vi "单道符合.vi"() -> ()   [LabVIEW 2014]
panel:
  in  "清零":bool
  in  "开始":bool
  out "状态":enum16{"初始化", "空闲", "配置", "读取", "退出"}(ring)
  out "coincnt":i32
  out "Bcnt":i32
  out "Acnt":i32
  in  "单道2道宽":u16=3000
  in  "单道2阈值电压":u16=100
  in  "单道1道宽":u16=3000
  in  "单道1阈值电压":u16=100
  in  "runtime(秒)":u16=10
  in  "cointime3":u16
  in  "cointime2":u16
  in  "cointime1":u16
  in  "退出":bool
  in  "读取":bool
  in  "配置":bool
  in  "初始状态":enum16{"初始化", "空闲", "配置", "读取", "退出"}(ring)
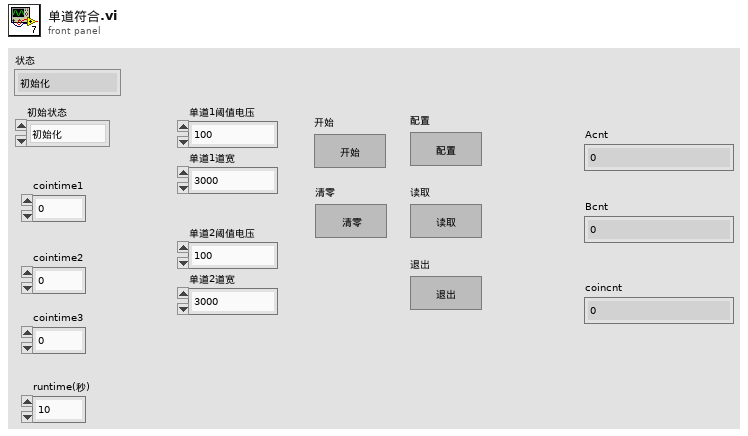
[diagram p1: front panel]
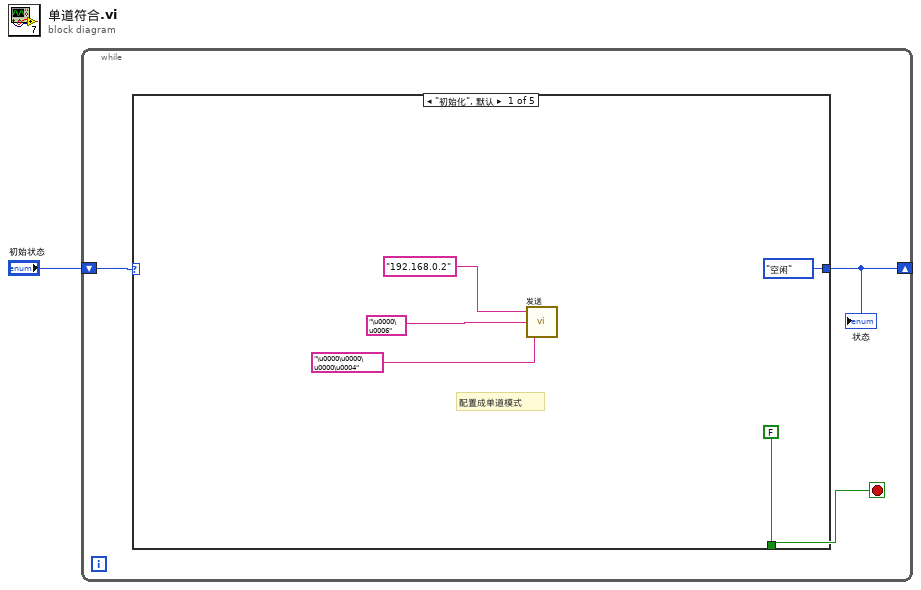
[diagram p0: block diagram]
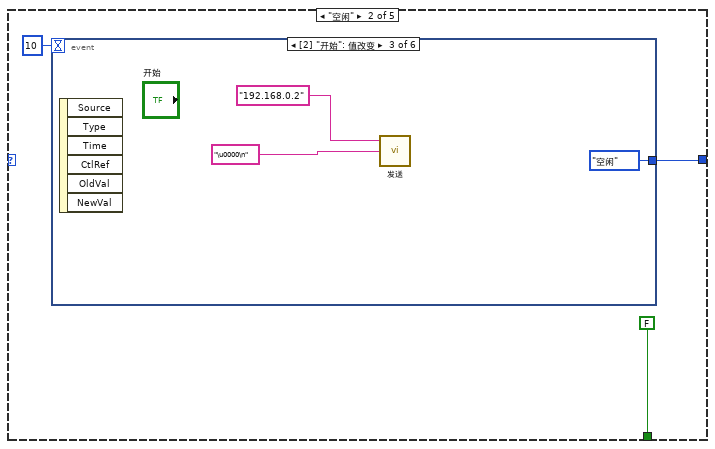
[diagram p2: hidden frame]
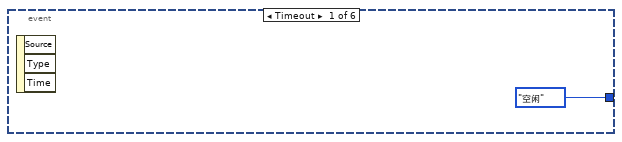
[diagram p3: hidden frame]
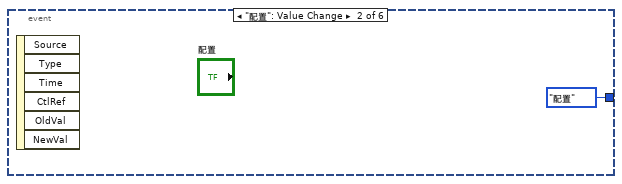
[diagram p4: hidden frame]
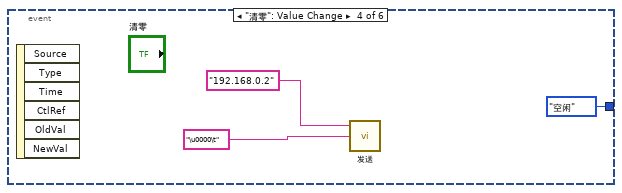
[diagram p5: hidden frame]
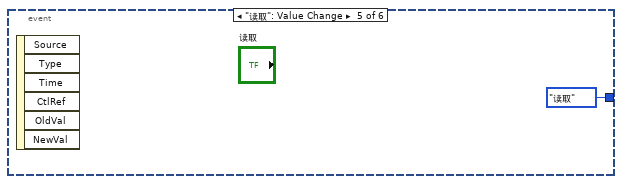
[diagram p6: hidden frame]
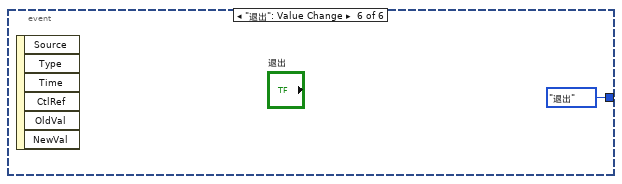
[diagram p7: hidden frame]
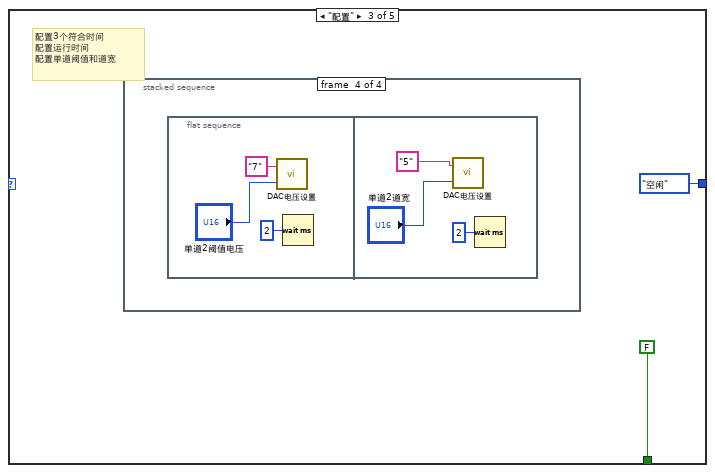
[diagram p8: hidden frame]
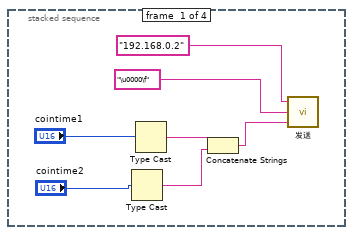
[diagram p9: hidden frame]
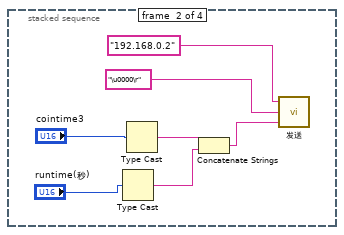
[diagram p10: hidden frame]
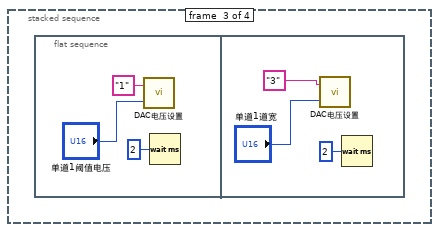
[diagram p11: hidden frame]
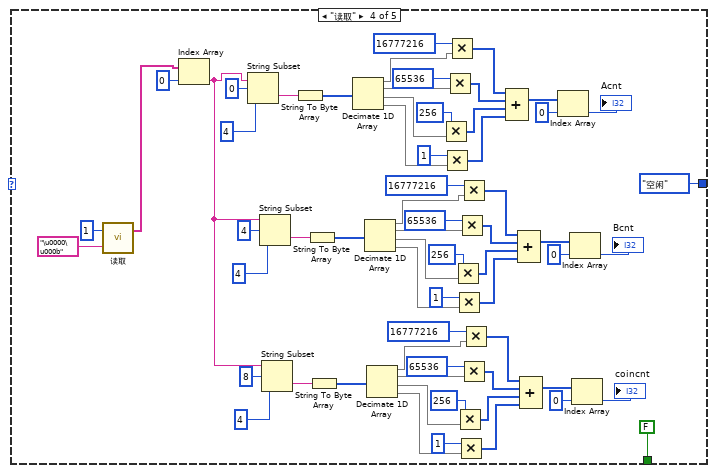
[diagram p12: hidden frame]
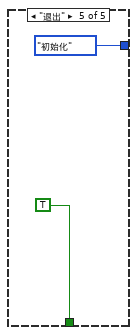
[diagram p13: hidden frame]
diagram:
  n1 = while {
    shift-right: [w3] -> _
    shift-left: "初始状态" -> [w4]
    stop <- w2 stop-if-true
    n2 = case shown="\"初始化\", 默认" w4 {
      tunnel: [enum16{"初始化", "空闲", "配置", "读取", "退出"}."空闲" ("初始状态") w11 enum16{"初始化", "空闲", "配置", "读取", "退出"}."空闲" ("初始状态") enum16{"初始化", "空闲", "配置", "读取", "退出"}."空闲" ("初始状态") enum16{"初始化", "空闲", "配置", "读取", "退出"}."初始化" ("初始状态")] -> w3
      tunnel: [FALSE FALSE FALSE FALSE TRUE] -> w2
      frame "初始化", Default {
        # "配置成单道模式"
        n3 = call "发送.vi"("数据（32bit）"="\u0000\u0000\u0000\u0004", "命令(16bit)"="\u0000\u0006", "目标IP"="192.168.0.2") -> ()  [unwired: 1 out]
      }
      frame "空闲" {
        n4 = event shown="[2] \"开始\": 值改变" {
          selector: _ -> [_ _ _ _ _ _]
          dyn-events: _ -> [_ _ _ _ _ _]
          timeout: 10 -> [_ _ _ _ _ _]
          tunnel: [enum16{"初始化", "空闲", "配置", "读取", "退出"}."空闲" ("初始状态") enum16{"初始化", "空闲", "配置", "读取", "退出"}."配置" ("初始状态") enum16{"初始化", "空闲", "配置", "读取", "退出"}."空闲" ("初始状态") enum16{"初始化", "空闲", "配置", "读取", "退出"}."空闲" ("初始状态") enum16{"初始化", "空闲", "配置", "读取", "退出"}."读取" ("初始状态") enum16{"初始化", "空闲", "配置", "读取", "退出"}."退出" ("初始状态")] -> w11
          event Timeout {
            n5 = event-data() -> ()  [unwired: 1 in, 3 out]
          }
          event "配置": Value Change {
            n6 = event-data() -> ()  [unwired: 1 in, 6 out]
          }
          event "开始": Value Change {
            n7 = event-data() -> ()  [unwired: 1 in, 6 out]
            n8 = call "发送.vi"("命令(16bit)"="\u0000\n", "目标IP"="192.168.0.2") -> ()  [unwired: 1 in, 1 out]
          }
          event "清零": Value Change {
            n9 = event-data() -> ()  [unwired: 1 in, 6 out]
            n10 = call "发送.vi"("命令(16bit)"="\u0000\t", "目标IP"="192.168.0.2") -> ()  [unwired: 1 in, 1 out]
          }
          event "读取": Value Change {
            n11 = event-data() -> ()  [unwired: 1 in, 6 out]
          }
          event "退出": Value Change {
            n12 = event-data() -> ()  [unwired: 1 in, 6 out]
          }
        }
      }
      frame "配置" {
        # "配置3个符合时间\n配置运行时间\n配置单道阈值和道宽"
        n13 = stacked-sequence {
          frame #0 {
            n14 = Type Cast(x="cointime2") -> (*(type *) &x=w27:string)  [unwired: 1 in]
            n15 = Type Cast(x="cointime1") -> (*(type *) &x=w28:string)  [unwired: 1 in]
            n16 = Concatenate Strings(w28, w27) -> (w29:string)
            n17 = call "发送.vi"("数据（32bit）"=w29, "命令(16bit)"="\u0000\f", "目标IP"="192.168.0.2") -> ()  [unwired: 1 out]
          }
          frame #1 {
            n18 = Type Cast(x="runtime(秒)") -> (*(type *) &x=w34:string)  [unwired: 1 in]
            n19 = Type Cast(x="cointime3") -> (*(type *) &x=w35:string)  [unwired: 1 in]
            n20 = Concatenate Strings(w35, w34) -> (w36:string)
            n21 = call "发送.vi"("数据（32bit）"=w36, "命令(16bit)"="\u0000\r", "目标IP"="192.168.0.2") -> ()  [unwired: 1 out]
          }
          frame #2 {
            n22 = flat-sequence {
              frame #0 {
                n23 = call "DAC电压设置.vi"("电压"="单道1阈值电压", "cmd_channel(8bit)"="1") -> ()  [unwired: 1 in]
                n24 = Wait (ms)(milliseconds to wait=u32 2 ("等待时间（毫秒）")) -> ()  [unwired: 1 out]
              }
              frame #1 {
                n25 = call "DAC电压设置.vi"("电压"="单道1道宽", "cmd_channel(8bit)"="3") -> ()  [unwired: 1 in]
                n26 = Wait (ms)(milliseconds to wait=u32 2 ("等待时间（毫秒）")) -> ()  [unwired: 1 out]
              }
            }
          }
          frame #3 {
            n27 = flat-sequence {
              frame #0 {
                n28 = call "DAC电压设置.vi"("电压"="单道2阈值电压", "cmd_channel(8bit)"="7") -> ()  [unwired: 1 in]
                n29 = Wait (ms)(milliseconds to wait=u32 2 ("等待时间（毫秒）")) -> ()  [unwired: 1 out]
              }
              frame #1 {
                n30 = call "DAC电压设置.vi"("电压"="单道2道宽", "cmd_channel(8bit)"="5") -> ()  [unwired: 1 in]
                n31 = Wait (ms)(milliseconds to wait=u32 2 ("等待时间（毫秒）")) -> ()  [unwired: 1 out]
              }
            }
          }
        }
      }
      frame "读取" {
        n32 = call "读取.vi"("命令"="\u0000\u000b", "帧数"=1) -> ("数组"=w92:string[])  [unwired: 1 out]
        n33 = Index Array(array=w92, index=0 ("索引")) -> (element=w51:string)
        n34 = String Subset(string=w51, offset (0)=0 ("偏移量(0)"), length (rest)=4 ("长度（剩余）")) -> (substring=w97:string)
        n35 = String Subset(string=w51, offset (0)=4 ("偏移量(0)"), length (rest)=4 ("长度（剩余）")) -> (substring=w77:string)
        n36 = String Subset(string=w51, offset (0)=8 ("偏移量(0)"), length (rest)=4 ("长度（剩余）")) -> (substring=w56:string)
        n37 = String To Byte Array(string=w97) -> (unsigned byte array=w96:u8[])
        n38 = String To Byte Array(string=w77) -> (unsigned byte array=w76:u8[])
        n39 = String To Byte Array(string=w56) -> (unsigned byte array=w55:u8[])
        n40 = Decimate 1D Array(w96) -> (w98:u8[], w99:u8[], w109:u8[], w108:u8[])
        n41 = Decimate 1D Array(w76) -> (w78:u8[], w79:u8[], w89:u8[], w88:u8[])
        n42 = Decimate 1D Array(w55) -> (w57:u8[], w58:u8[], w68:u8[], w67:u8[])
        n43 = Multiply(x=256, y=w109) -> (x*y=w104:i32[])
        n44 = Multiply(x=1, y=w108) -> (x*y=w105:i32[])
        n45 = Multiply(x=65536, y=w99) -> (x*y=w101:i32[])
        n46 = Multiply(x=16777216, y=w98) -> (x*y=w100:i32[])
        n47 = Multiply(x=256, y=w89) -> (x*y=w84:i32[])
        n48 = Multiply(x=1, y=w88) -> (x*y=w85:i32[])
        n49 = Multiply(x=256, y=w68) -> (x*y=w63:i32[])
        n50 = Multiply(x=1, y=w67) -> (x*y=w64:i32[])
        n51 = Multiply(x=65536, y=w79) -> (x*y=w81:i32[])
        n52 = Multiply(x=16777216, y=w78) -> (x*y=w80:i32[])
        n53 = Multiply(x=65536, y=w58) -> (x*y=w60:i32[])
        n54 = Multiply(x=16777216, y=w57) -> (x*y=w59:i32[])
        n55 = Compound Arithmetic op=ADD(w100, w101, w104, w105) -> (w95:i32[])
        n56 = Compound Arithmetic op=ADD(w80, w81, w84, w85) -> (w75:i32[])
        n57 = Compound Arithmetic op=ADD(w59, w60, w63, w64) -> (w54:i32[])
        n58 = Index Array(array=w95, index=0 ("索引")) -> (element=→"Acnt":i32)
        n59 = Index Array(array=w75, index=0 ("索引")) -> (element=→"Bcnt":i32)
        n60 = Index Array(array=w54, index=0 ("索引")) -> (element=→"coincnt":i32)
      }
      frame "退出" {
      }
    }
    "状态" <- w3
  }
